vi "Generate Value.vi"(8 "error in (no error)":errorcluster, 10 "base value":i64, 11 "value in":refnum<class "NT Base.lvclass">) -> (0 "error out":errorcluster, 3 "value out":refnum<class "NT Base.lvclass">)   [LabVIEW 2020, in "PV Access.lvlib" / "PV Data.lvlib"]
uses:
  PV Data.lvlib
  NT Base/NT Base.lvclass
  NT Scalar/NT Scalar.lvclass
  C:/Users/eyw68381/source/repos/pvaccess-labview/labview/source/PV Data/NT Base/NT Base.lvclass
  NT Enum/NT Enum.lvclass
  3336d5e6-6b46-40cc-8581-c00a96048cf3.vi
  c0315305-4ea9-43e2-99a8-a5923f228944.vi
  e9ef65dd-4b85-465f-aa80-4b18505edb13.vi
  babcc117-bc44-41a1-9c2b-73189d1bbfcb.vi
  c68d18eb-9334-419f-972f-f5b5be29402e.vi
  54e220c7-dbf9-4865-aabc-812fe05ebb8b.vi
  47823474-13c3-4f35-a55b-4dd444e3f7d9.vi
  e6de0aaa-8fd3-4213-bbd6-031fb177ed83.vi
  115dbf5b-fdea-438f-8eda-7315cadb6382.vi
  228aee6f-7479-4422-86e8-739061133d5f.vi
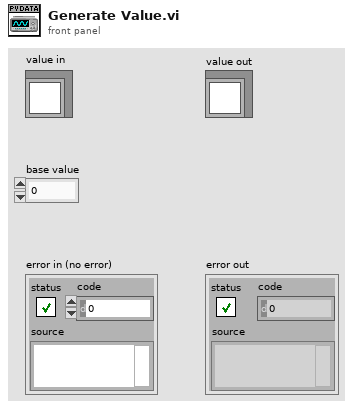
[diagram p1: front panel]
types:
  T1 = typedef "PV Access.lvlib/PV Data.lvlib/Type Code.ctl" = enum8{"Null", "Bool", "BoolA", "Int8", "Int8A", "Int16", "Int16A", "Int32", "Int32A", "Int64", "Int64A", "UInt8", "UInt8A", "UInt16", "UInt16A", "UInt32", "UInt32A", "UInt64", "UInt64A", "Float32", "Float32A", "Float64", "Float64A", "String", "StringA", "Struct", "StructA", "Union", "UnionA", "Any", "AnyA"}
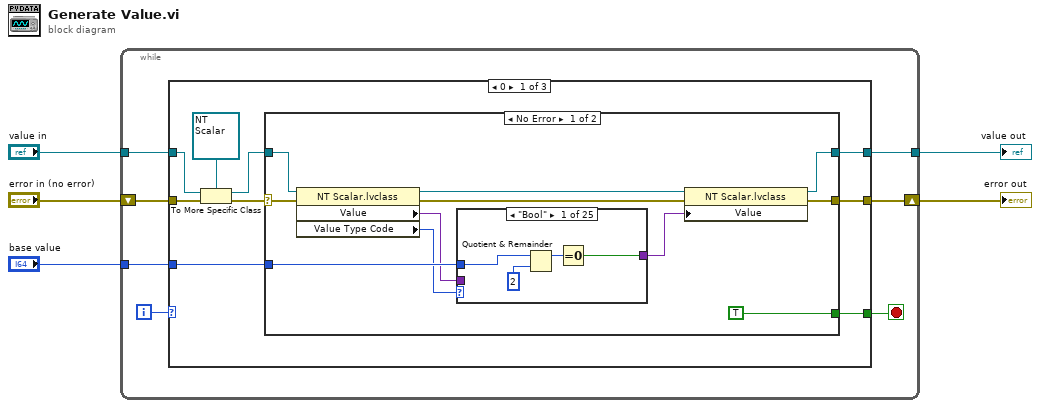
[diagram p0: block diagram]
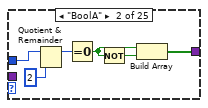
[diagram p2: hidden frame]
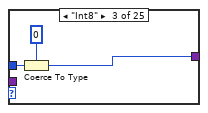
[diagram p3: hidden frame]
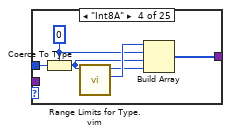
[diagram p4: hidden frame]
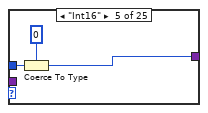
[diagram p5: hidden frame]
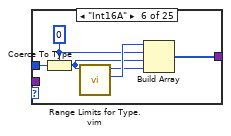
[diagram p6: hidden frame]
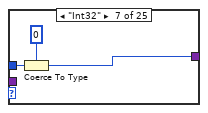
[diagram p7: hidden frame]
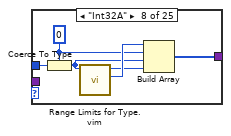
[diagram p8: hidden frame]
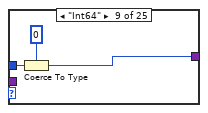
[diagram p9: hidden frame]
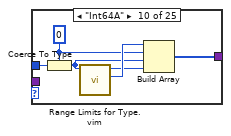
[diagram p10: hidden frame]
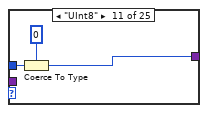
[diagram p11: hidden frame]
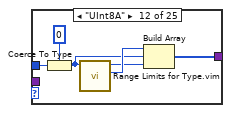
[diagram p12: hidden frame]
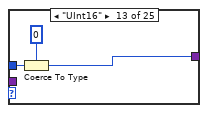
[diagram p13: hidden frame]
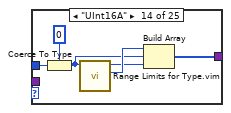
[diagram p14: hidden frame]
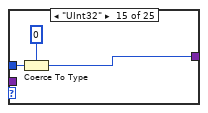
[diagram p15: hidden frame]
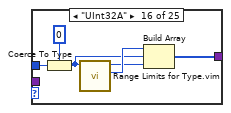
[diagram p16: hidden frame]
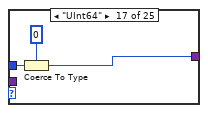
[diagram p17: hidden frame]
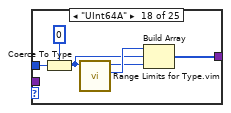
[diagram p18: hidden frame]
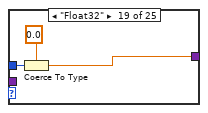
[diagram p19: hidden frame]
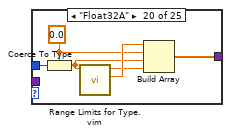
[diagram p20: hidden frame]
diagram:
  n1 = while {
    tunnel: "base value" -> [w12]
    tunnel: [w11] -> w4
    tunnel: "value in" -> [w8]
    shift-right: [w9] -> w2
    shift-left: "error in (no error)" -> [w10]
    i -> [w7]
    stop <- w6 stop-if-true
    n2 = case shown="0" w7 {
      tunnel: w12 -> [w21 w152 _]
      tunnel: [w20 w151 w170] -> w11
      tunnel: w10 -> [w14 w145 w169]
      tunnel: [w19 w150 w169] -> w9
      tunnel: w8 -> [w18 w149 w170]
      tunnel: [w13 w144 TRUE] -> w6
      frame 0 {
        n3 = To More Specific Class(target class=refnum<class "NT Scalar.lvclass"> refnum ("PV Access.lvlib:PV Data.lvlib:NT Scalar.lvclass"), reference=w18, error in=w14) -> (specific class reference=w15:refnum<class "NT Scalar.lvclass">, error out=w16:errorcluster)
        n4 = case shown="No Error" w16 {
          selector: w16 -> [w31 w142]
          tunnel: w21 -> [w32 _]
          tunnel: [w23 w143] -> w20
          tunnel: [w24 w141] -> w19
          tunnel: w15 -> [w30 w143]
          tunnel: [TRUE _] -> w13
          frame No Error {
            n5 = property class="NT Scalar.lvclass"(reference=w30, error in=w31) -> (reference out=w26:refnum<class "NT Scalar.lvclass">, error out=w27:errorcluster, "Value"=w28:variant, "Value Type Code"=w29:T1)
            n6 = case shown="\"Bool\"" w29 {
              tunnel: w32 -> [w35 w40 w44 w51 w53 w60 w62 w69 w71 w78 w80 w87 w89 w96 w98 w105 w107 w114 w116 w123 w125 w132 w134 w138 _]
              tunnel: [w34 w42 w43 w50 w52 w59 w61 w68 w70 w77 w79 w86 w88 w95 w97 w104 w106 w113 w115 w122 w124 w131 w133 w135 w139] -> w25
              tunnel: w28 -> [_ _ _ _ _ _ _ _ _ _ _ _ _ _ _ _ _ _ _ _ _ _ _ _ w139]
              frame "Bool" {
                n7 = Quotient & Remainder(x=w35, y=i64 2) -> (x-y*floor(x/y)=w33:i64)  [unwired: 1 out]
                n8 = Equal To 0?(x=w33) -> (x = 0?=w34:bool)
              }
              frame "BoolA" {
                n9 = Quotient & Remainder(x=w40, y=i64 2) -> (x-y*floor(x/y)=w39:i64)  [unwired: 1 out]
                n10 = Equal To 0?(x=w39) -> (x = 0?=w37:bool)
                n11 = Not(x=w37) -> (.not. x?=w38:bool)
                n12 = Build Array(w37, w38) -> (w42:bool[])
              }
              frame "Int8" {
                n13 = Coerce To Type(0:w44, 1:i8 0 ("default value")) -> (2:w43:i8)
              }
              frame "Int8A" {
                w47 = i8 0 ("default value")
                n14 = Coerce To Type(0:w51, 1:w47) -> (2:w46:i8)
                n15 = call "Range Limits for Type.vim"("type"=w46) -> ("minimum value for type"=w49:i8, "maximum value for type"=w48:i8)  [unwired: 9 in]
                n16 = Build Array(w49, w47, w46, w48) -> (w50:i8[])
              }
              frame "Int16" {
                n17 = Coerce To Type(0:w53, 1:i16 0 ("default value")) -> (2:w52:i16)
              }
              frame "Int16A" {
                w56 = i16 0 ("default value")
                n18 = Coerce To Type(0:w60, 1:w56) -> (2:w55:i16)
                n19 = call "Range Limits for Type.vim"("type"=w55) -> ("minimum value for type"=w58:i16, "maximum value for type"=w57:i16)  [unwired: 9 in]
                n20 = Build Array(w58, w56, w55, w57) -> (w59:i16[])
              }
              frame "Int32" {
                n21 = Coerce To Type(0:w62, 1:0 ("default value")) -> (2:w61:i32)
              }
              frame "Int32A" {
                w65 = 0 ("default value")
                n22 = Coerce To Type(0:w69, 1:w65) -> (2:w64:i32)
                n23 = call "Range Limits for Type.vim"("type"=w64) -> ("minimum value for type"=w67:i32, "maximum value for type"=w66:i32)  [unwired: 9 in]
                n24 = Build Array(w67, w65, w64, w66) -> (w68:i32[])
              }
              frame "Int64" {
                n25 = Coerce To Type(0:w71, 1:i64 0 ("default value")) -> (2:w70:i64)
              }
              frame "Int64A" {
                w74 = i64 0 ("default value")
                n26 = Coerce To Type(0:w78, 1:w74) -> (2:w73:i64)
                n27 = call "Range Limits for Type.vim"("type"=w73) -> ("minimum value for type"=w76:i64, "maximum value for type"=w75:i64)  [unwired: 9 in]
                n28 = Build Array(w76, w74, w73, w75) -> (w77:i64[])
              }
              frame "UInt8" {
                n29 = Coerce To Type(0:w80, 1:u8 0 ("default value")) -> (2:w79:u8)
              }
              frame "UInt8A" {
                n30 = Coerce To Type(0:w87, 1:u8 0 ("default value")) -> (2:w83:u8)
                n31 = call "Range Limits for Type.vim"("type"=w83) -> ("minimum value for type"=w85:u8, "maximum value for type"=w82:u8)  [unwired: 9 in]
                n32 = Build Array(w85, w83, w82) -> (w86:u8[])
              }
              frame "UInt16" {
                n33 = Coerce To Type(0:w89, 1:u16 0 ("default value")) -> (2:w88:u16)
              }
              frame "UInt16A" {
                n34 = Coerce To Type(0:w96, 1:u16 0 ("default value")) -> (2:w92:u16)
                n35 = call "Range Limits for Type.vim"("type"=w92) -> ("minimum value for type"=w94:u16, "maximum value for type"=w91:u16)  [unwired: 9 in]
                n36 = Build Array(w94, w92, w91) -> (w95:u16[])
              }
              frame "UInt32" {
                n37 = Coerce To Type(0:w98, 1:u32 0 ("default value")) -> (2:w97:u32)
              }
              frame "UInt32A" {
                n38 = Coerce To Type(0:w105, 1:u32 0 ("default value")) -> (2:w101:u32)
                n39 = call "Range Limits for Type.vim"("type"=w101) -> ("minimum value for type"=w103:u32, "maximum value for type"=w100:u32)  [unwired: 9 in]
                n40 = Build Array(w103, w101, w100) -> (w104:u32[])
              }
              frame "UInt64" {
                n41 = Coerce To Type(0:w107, 1:u64 0 ("default value")) -> (2:w106:u64)
              }
              frame "UInt64A" {
                n42 = Coerce To Type(0:w114, 1:u64 0 ("default value")) -> (2:w110:u64)
                n43 = call "Range Limits for Type.vim"("type"=w110) -> ("minimum value for type"=w112:u64, "maximum value for type"=w109:u64)  [unwired: 9 in]
                n44 = Build Array(w112, w110, w109) -> (w113:u64[])
              }
              frame "Float32" {
                n45 = Coerce To Type(0:w116, 1:sgl 0.0 ("default value")) -> (2:w115:sgl)
              }
              frame "Float32A" {
                w119 = sgl 0.0 ("default value")
                n46 = Coerce To Type(0:w123, 1:w119) -> (2:w118:sgl)
                n47 = call "Range Limits for Type.vim"("type"=w118) -> ("minimum value for type"=w121:sgl, "maximum value for type"=w120:sgl)  [unwired: 9 in]
                n48 = Build Array(w121, w119, w118, w120) -> (w122:sgl[])
              }
              frame "Float64" {
                n49 = Coerce To Type(0:w125, 1:0.0 ("default value")) -> (2:w124:dbl)
              }
              frame "Float64A" {
                w128 = 0.0 ("default value")
                n50 = Coerce To Type(0:w132, 1:w128) -> (2:w127:dbl)
                n51 = call "Range Limits for Type.vim"("type"=w127) -> ("minimum value for type"=w130:dbl, "maximum value for type"=w129:dbl)  [unwired: 9 in]
                n52 = Build Array(w130, w128, w127, w129) -> (w131:dbl[])
              }
              frame "String" {
                n53 = Format Value(value (0)=w134) -> (output string=w133:string)  [unwired: 2 in]
              }
              frame "StringA" {
                n54 = Format Value(value (0)=w138) -> (output string=w137:string)  [unwired: 2 in]
                n55 = Build Array(w137, "Hello" ("element")) -> (w135:string[])
              }
              frame Default {
              }
            }
            n56 = property class="NT Scalar.lvclass"(reference=w26, error in=w27, "Value"=w25) -> (reference out=w23:refnum<class "NT Scalar.lvclass">, error out=w24:errorcluster)
          }
          frame Error {
            n57 = call <vilib>:"Clear Errors.vi"("error in (no error)"=w142, "specific error code to clear (0: all)"=1448) -> ("error out"=w141:errorcluster)  [unwired: 4 in, 1 out]
          }
        }
      }
      frame 1 {
        n58 = To More Specific Class(target class=refnum<class "NT Enum.lvclass"> refnum ("PV Access.lvlib:PV Data.lvlib:NT Enum.lvclass"), reference=w149, error in=w145) -> (specific class reference=w146:refnum<class "NT Enum.lvclass">, error out=w147:errorcluster)
        n59 = case shown="Error .." w147 {
          selector: w147 -> [w163 w166]
          tunnel: w152 -> [w154 _]
          tunnel: [w158 w167] -> w151
          tunnel: [w159 w165] -> w150
          tunnel: w146 -> [w162 w167]
          tunnel: [TRUE _] -> w144
          frame No Error {
            n60 = property class="NT Enum.lvclass"(reference=w162, error in=w163) -> (reference out=w160:refnum<class "NT Enum.lvclass">, error out=w161:errorcluster, "Choices"=w156:string[])
            n61 = Array Size(array=w156) -> (size(s)=w155:i32)
            n62 = Quotient & Remainder(x=w154, y=w155) -> (x-y*floor(x/y)=w153:i64)  [unwired: 1 out]
            n63 = property class="NT Enum.lvclass"(reference=w160, error in=w161, "Index"=w153) -> (reference out=w158:refnum<class "NT Enum.lvclass">, error out=w159:errorcluster)
          }
          frame Error {
            n64 = call <vilib>:"Clear Errors.vi"("error in (no error)"=w166, "specific error code to clear (0: all)"=1448) -> ("error out"=w165:errorcluster)  [unwired: 4 in, 1 out]
          }
        }
      }
      frame Default {
      }
    }
  }
  "value out" <- w4
  "error out" <- w2
